vi "hReadChannels-UandP-2013.vi"(4 "RawScal":sgl[](array[numeric]), 5 "SumScal":sgl[](array[numeric]), 6 "Scale(mV)":sgl[](array[numeric]), 7 "Tau/dt":sgl[](array[numeric]), 8 "error in":errorcluster, 9 "Nsamples":u32, 11 "FPGA VI Reference In":refnum<k20>) -> (0 "error out":errorcluster, 1 "RawArray":sgl[][](array[numeric]), 2 "PowerArray":sgl[][](array[numeric]), 3 "FPGA VI Reference Out":refnum<k20>, 10 "Fehler":bool)   [LabVIEW 2014]
doc: "startet das einlesen und führt dies bis n Samples aus\nHier mit FIFO und IRQ."
uses:
  <vilib>/Utility/error.llb/Error Cluster From Error Code.vi
  <vilib>/rvi/errors/niLvFpgaAdjustHostInterfaceError.vi
  <vilib>/RVI Host/nirviSupport.llb/nirviErrorClusterFromErrorCode.vi
  <vilib>/rvi/interface/nirviReadWriteControl/nirviReadWriteControl.xnode
  FPGA Bitfiles/W7XBolo2017_FPGATarget_FlorianDefault.lvbitx
  f_main_2014.vi
  <vilib>/rvi/interface/nirviMethod/nirviMethod.xnode
  NiFpgaLv.dll
  <vilib>/rvi/interface/nirviMethod/StockFPGA_InlinedMethodWaitForMultipleIRQ.vi
  <vilib>/FPGAPlugInAG/PCI-7813R/niLvFpga_WaitOnIrq_PCI-7813R.vi
  <vilib>/FPGAPlugInAG/PCI-7813R/niLvFpga_AcknowledgeIrq_PCI-7813R.vi
  <vilib>/FPGAPlugInAG/PCI-7813R/niLvFpga_ReadFifo_PCI-7813R.vi
  <vilib>/rvi/errors/niLvFpgaMergeErrorWithErrorCode.vi
panel:
  out "Elements Remaining":u32
  out "STOP?":bool
  out "Timed Out":bool
  # "Sampling"
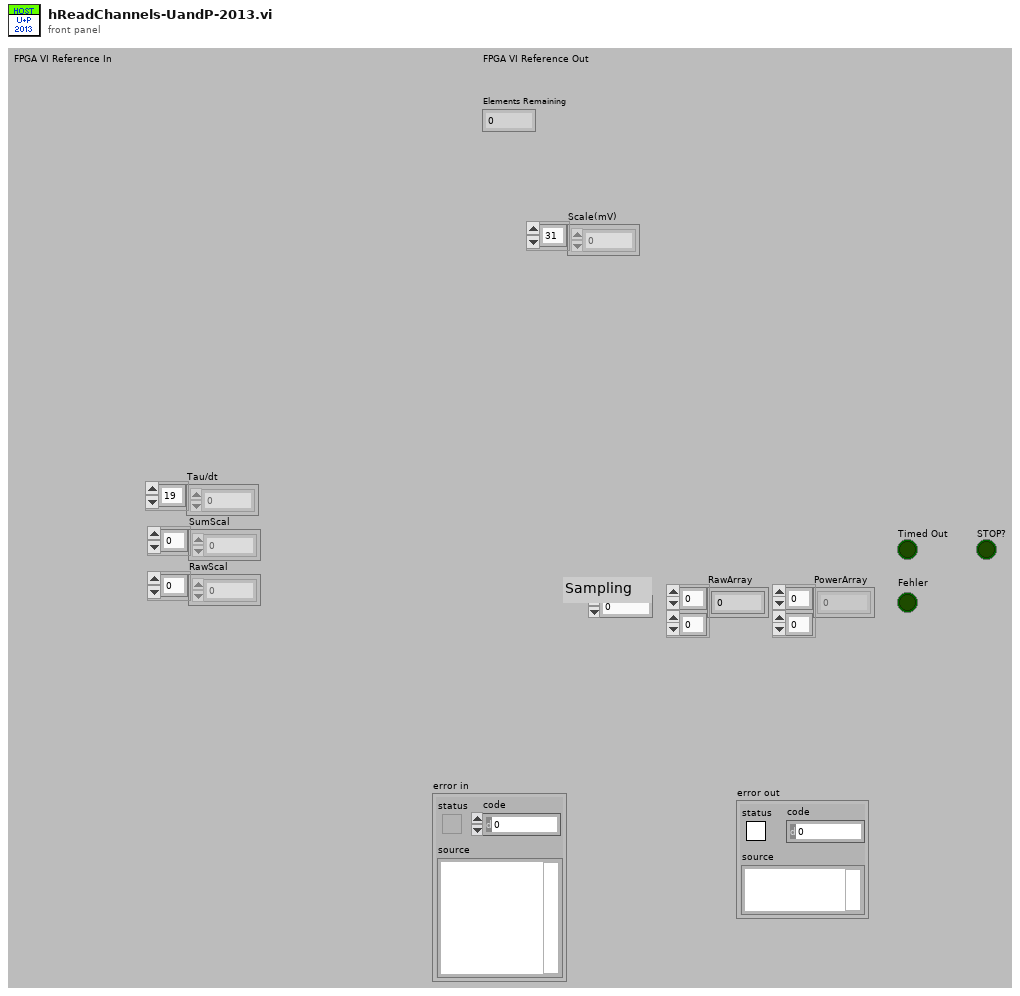
[diagram p1: front panel]
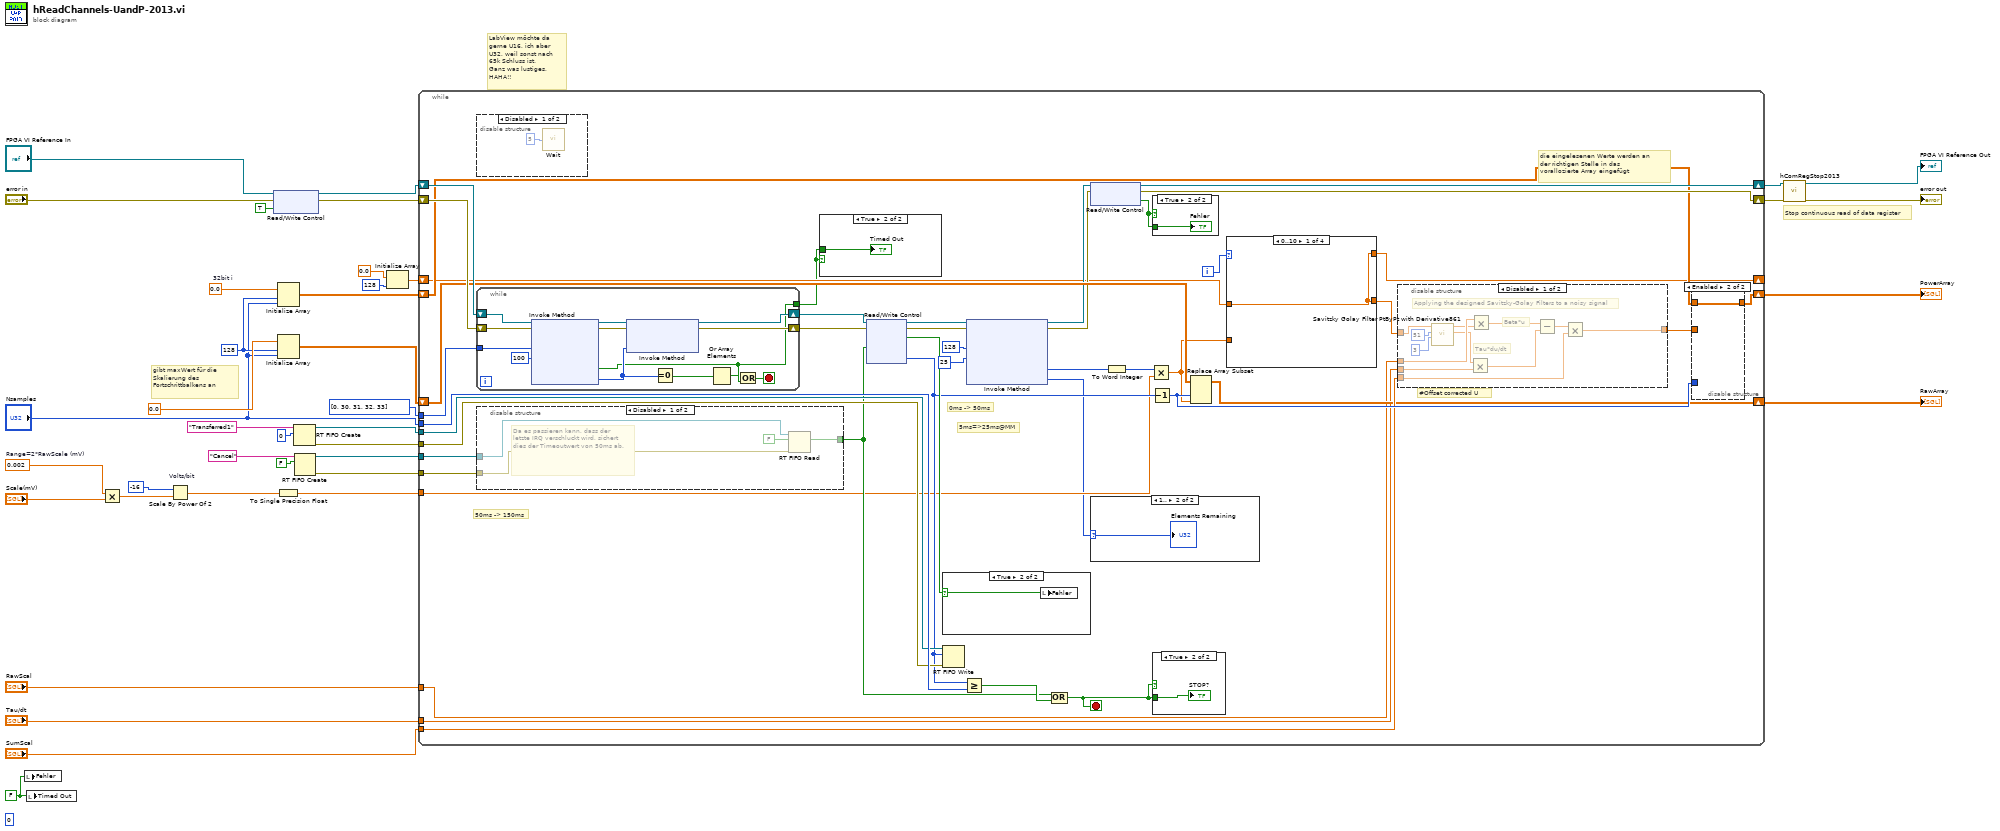
[diagram p0: block diagram]
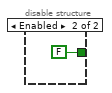
[diagram p4: hidden frame]
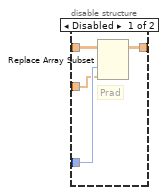
[diagram p5: hidden frame]
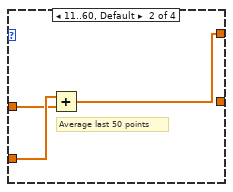
[diagram p10: hidden frame]
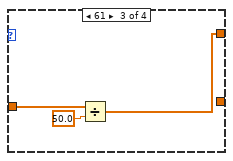
[diagram p11: hidden frame]
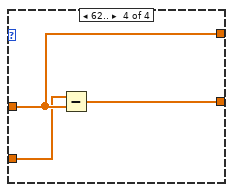
[diagram p12: hidden frame]
diagram:
  w11 = 0.002  # Range=2*RawScale (mV)
  (unwired) 0
  w21 = 128 ("dimension size")
  w31 = sgl 0.0  # 32bit i
  w29 = FALSE
  # "Stop continuous read of data register"
  # "gibt maxWert für die Skalierung des Fortschrittbalkens an"
  # "LabView möchte da gerne U16, ich aber U32, weil sonst nach 65k Schluss ist. \nGanz was lustiges, HAHA!!"
  n1 = local write "Fehler"(w29) -> ()
  n2 = local write "Timed Out"(w29) -> ()
  n3 = Multiply(x=w11, y="Scale(mV)") -> (x*y=w12:dbl[])
  n4 = Scale By Power Of 2 "Volts/bit"(n=i16 -16, x=w12) -> (x*2^n=w13:dbl[])
  n5 = xnode "Read/Write Control"("FPGA VI Reference In"="FPGA VI Reference In", "error in"="error in", "ADCRead"=TRUE) -> ("FPGA VI Reference Out"=w17:refnum<k20>, "error out"=w16:errorcluster)
  n6 = Initialize Array(w31, w21, "Nsamples") -> (w30:sgl[][])
  n7 = Initialize Array(sgl 0.0, w21, "Nsamples") -> (w39:sgl[][])
  n8 = To Single Precision Float(number=w13) -> (single precision float=w10:sgl[])
  n9 = RT FIFO Create(0:"Transferred1" ("name (unnamed)"), 1:u32 0) -> (8:w36:refnum<k33>, 11:w35:errorcluster)  [unwired: 2 in, 5 out]
  n10 = RT FIFO Create(0:"Cancel" ("name (unnamed)"), 1:FALSE) -> (8:w33:refnum<k33>, 11:w32:errorcluster)  [unwired: 2 in, 5 out]
  n11 = Initialize Array(sgl 0.0 ("element"), 128 ("dimension size")) -> (w3:sgl[])
  n12 = while {
    tunnel: "Nsamples" -> [w77]
    shift-right: [w60] -> w22
    shift-left: w39 -> [w66]
    shift-right: [w78] -> w28
    shift-left: w17 -> [w81]
    shift-right: [w79] -> w27
    shift-left: w16 -> [w80]
    tunnel: w36 -> [w76]
    tunnel: w35 -> [w75]
    tunnel: w33 -> [w73]
    tunnel: w32 -> [w72]
    shift-right: [w70] -> w23
    shift-left: w30 -> [w71]
    tunnel: w10 -> [w63]
    tunnel: "Tau/dt" -> [w58]
    tunnel: "SumScal" -> [w61]
    tunnel: "RawScal" -> [w59]
    shift-right: [w49] -> _
    shift-left: w3 -> [w48]
    tunnel: i32[] [0, 30, 31, 32, 33] -> [w42]
    i -> [w62]
    stop <- w43 stop-if-true
    # "5ms=>25ms@MM"
    # "0ms -> 50ms"
    # "50ms -> 150ms"
    # "#Offset corrected U"
    # "die eingelesenen Werte werden an der richtigen Stelle in das vorallozierte Array eingefügt"
    n13 = disable-structure shown="Disabled" {
      frame Disabled {
        n14 = call "Wait"("Count(uSec)"=u32 5) -> ()  [unwired: 1 out]
      }
      frame Enabled {
      }
    }
    n15 = while {
      tunnel: [w86] -> w46
      shift-right: [w88] -> w40
      shift-left: w81 -> [w95]
      shift-right: [w87] -> w41
      shift-left: w80 -> [w94]
      tunnel: w42 -> [w92]
      stop <- w85 stop-if-true
      n16 = xnode "Invoke Method"("FPGA VI Reference In"=w95, "error in"=w94, "IRQ Number(s)"=w92, "Timeout (ms)"=100) -> ("FPGA VI Reference Out"=w89:refnum<k20>, "error out"=w90:errorcluster, "Timed Out"=w86:bool, "IRQ(s) Asserted"=w91:i32[])
      n17 = xnode "Invoke Method"("FPGA VI Reference In"=w89, "error in"=w90, "IRQ Number(s)"=w91) -> ("FPGA VI Reference Out"=w88:refnum<k20>, "error out"=w87:errorcluster)
      n18 = Equal To 0?(x=w91) -> (x = 0?=w84:bool[])
      n19 = Or Array Elements(Boolean array=w84) -> (logical OR=w83:bool)
      n20 = Or(x=w83, y=w86) -> (x .or. y?=w85:bool)
    }
    n21 = disable-structure shown="Disabled" {
      disable-tunnel: [w101 FALSE] -> w74
      disable-tunnel: w73 -> [w100 _]
      disable-tunnel: w72 -> [w99 _]
      frame Disabled {
        # "Da es passieren kann, dass der letzte IRQ verschluckt wird, sichert dies der Timeoutwert von 50ms ab."
        n22 = RT FIFO Read(0:w100, 1:FALSE ("element"), 3:w99) -> (9:w101:bool)  [unwired: 5 out]
      }
      frame Enabled {
      }
    }
    n23 = case shown="True" w46 {
      tunnel: w46 -> [_ w109]
      frame False {
      }
      frame True {
        "Timed Out" <- w109
      }
    }
    n24 = xnode "Read/Write Control"("FPGA VI Reference In"=w40, "error in"=w41, "cancel"=w74) -> ("FPGA VI Reference Out"=w68:refnum<k20>, "error out"=w67:errorcluster, "Timeout"=w69:bool, "ScanID"=w64:u32)
    n25 = case shown="True" w69 {
      selector: w69 -> [_ w134]
      frame False {
      }
      frame True {
        n26 = local write "Fehler"(w134) -> ()
      }
    }
    n27 = RT FIFO Write(0:w76, 1:w64, 3:w75) -> ()  [unwired: 1 in, 5 out]
    n28 = Greater Or Equal?(x=w64, y=w77) -> (x >= y?=w82:bool)
    n29 = xnode ("Invoke Method")("FPGA VI Reference In"=w68, "error in"=w67, "Number of Elements"=u32 128, "Timeout (ms)"=25 ("Timeout")) -> ("FPGA VI Reference Out"=w52:refnum<k20>, "error out"=w51:errorcluster, "Data"=w55:u32[], "Elements Remaining"=w45:u32)
    n30 = Compound Arithmetic op=OR(w74, w82) -> (w43:bool)
    n31 = xnode "Read/Write Control"("FPGA VI Reference In"=w52, "error in"=w51) -> ("FPGA VI Reference Out"=w78:refnum<k20>, "error out"=w79:errorcluster, "Fifo-Fehler"=w44:bool)
    n32 = case shown="1.." w45 {
      selector: w45 -> [_ w108]
      frame 0, Default {
      }
      frame 1.. {
        "Elements Remaining" <- w108
      }
    }
    n33 = To Word Integer(number=w55) -> (16bit integer=w54:i16[])
    n34 = Multiply(x=w54, y=w63) -> (x*y=w50:sgl[])
    n35 = Decrement(x=w64) -> (x-1=w65:u32)
    n36 = case shown="True" w44 {
      tunnel: w44 -> [_ w97]
      frame False {
      }
      frame True {
        "Fehler" <- w97
      }
    }
    n37 = case shown="True" w43 {
      tunnel: w43 -> [_ w96]
      frame False {
      }
      frame True {
        "STOP?" <- w96
      }
    }
    n38 = Replace Array Subset(array=w66, new element=w50, index (col)=w65) -> (w60:sgl[][])  [unwired: 1 in]
    n39 = case shown="0..10" w62 {
      tunnel: w50 -> [_ w126 _ w132]
      tunnel: [w124 w127 w129 w133] -> w49
      tunnel: w48 -> [w124 w125 w130 w133]
      tunnel: [w124 _ _ w131] -> w47
      frame 0..10 {
      }
      frame 11..60, Default {
        # "Average last 50 points"
        n40 = Add(x=w126, y=w125) -> (x+y=w127:sgl[])
      }
      frame 61 {
        n41 = Divide(x=w130, y=sgl 50.0) -> (x/y=w129:sgl[])
      }
      frame 62.. {
        n42 = Subtract(x=w132, y=w133) -> (x-y=w131:sgl[])
      }
    }
    n43 = disable-structure shown="Disabled" {
      disable-tunnel: w61 -> [w121 _]
      disable-tunnel: w59 -> [w120 _]
      disable-tunnel: w58 -> [w119 _]
      disable-tunnel: [w118 w122] -> w53
      disable-tunnel: w47 -> [w117 w122]
      frame Disabled {
        # "Beta*u"
        # "Tau*du/dt"
        # "Applying the designed Savitzky-Golay Filters to a noisy signal"
        n44 = call "Savitzky Golay Filter PtByPt with Derivative861.vi"("order polynomial"=3, "side points"=51, "x"=w117) -> ("Filtered Derivative"=w113:dbl[], "Filtered x"=w114:dbl[])  [unwired: 1 in, 6 out]
        n45 = Multiply(x=w113, y=w119) -> (x*y=w112:dbl[])
        n46 = Multiply(x=w120, y=w114) -> (x*y=w116:dbl[])
        n47 = Subtract(x=w116, y=w112) -> (x-y=w115:dbl[])
        n48 = Multiply(x=w115, y=w121) -> (x*y=w118:dbl[])
      }
      frame Enabled {
      }
    }
    n49 = disable-structure shown="Enabled" {
      disable-tunnel: w71 -> [w106 w107]
      disable-tunnel: [w105 w107] -> w70
      disable-tunnel: w65 -> [w104 _]
      disable-tunnel: w53 -> [w103 _]
      frame Disabled {
        # "Prad"
        n50 = Replace Array Subset(array=w106, new element=w103, index (col)=w104) -> (w105:sgl[][])  [unwired: 1 in]
      }
      frame Enabled {
      }
    }
  }
  "RawArray" <- w22
  "PowerArray" <- w23
  n51 = call "hComRegStop2013.vi"("error in"=w27, "FPGA VI Reference In"=w28) -> ("error out"=→"error out":errorcluster, "FPGA VI Reference Out"=→"FPGA VI Reference Out":refnum<k20>)  [unwired: 3 in, 1 out]
